vi "HoppingStep(Nonlinear-XZEnhancedSampleCurr).vi"() -> ()   [LabVIEW 2014]
uses:
  <vilib>/Platform/TimedLoop/XDataNode/timing_clust.ctl
  <vilib>/Platform/TimedLoop/XDataNode/nitl_modes.ctl
  <vilib>/Platform/TimedLoop/XDataNode/wakeup.ctl
  <vilib>/rvi/Emulation/niFpgaGetClockAttributes.vi
  <vilib>/rvi/Emulation/niFpgaSctlEmulationGetInTimedLoop.vi
  <vilib>/rvi/Emulation/niFpgaEmulationReportErrorSimple.vi
  <vilib>/rvi/Emulation/niFpgaProcessEmulError.vi
  <vilib>/rvi/eio/common/nirviEmuTemplateMethod_errors.vi
  <vilib>/rvi/Emulation/niFpgaCriticalErrorInLSC.vi
  <vilib>/rvi/interface/RandomDataEmulation/niFpgaRandomDataHandleErrors.vi
  <vilib>/eio/EIONode/EIONode.xnode
  <vilib>/Platform/TimedLoop/XDataNode/XDataNode.xnode
  <vilib>/rvi/DataTransferAndStorage/Container/XNode/niFpgaContainer.xnode
  <vilib>/rvi/interface/RandomDataEmulation/nirviRandomDataFpgaReadWriteTemplate.vi
  <vilib>/Platform/TimedLoop/XDataNode/XDNodeRunTimeDep.lvlib
panel:
  in  "ZLimitFluctuationRange":i16
  in  "CheckNum":i16
  in  "BottomSleep us":i16=80
  in  "UpperSleep us":i16=150
  out "ZRealPos":i16
  in  "RelativeWithdraw":i16
  out "Waveform Chart":i32(graph)
  in  "stop":bool
  out "Z":i32(graph)
  in  "ZOffset":i16
  in  "XOffset":i16
  in  "XNum":i16
  in  "XStepIndex":i16
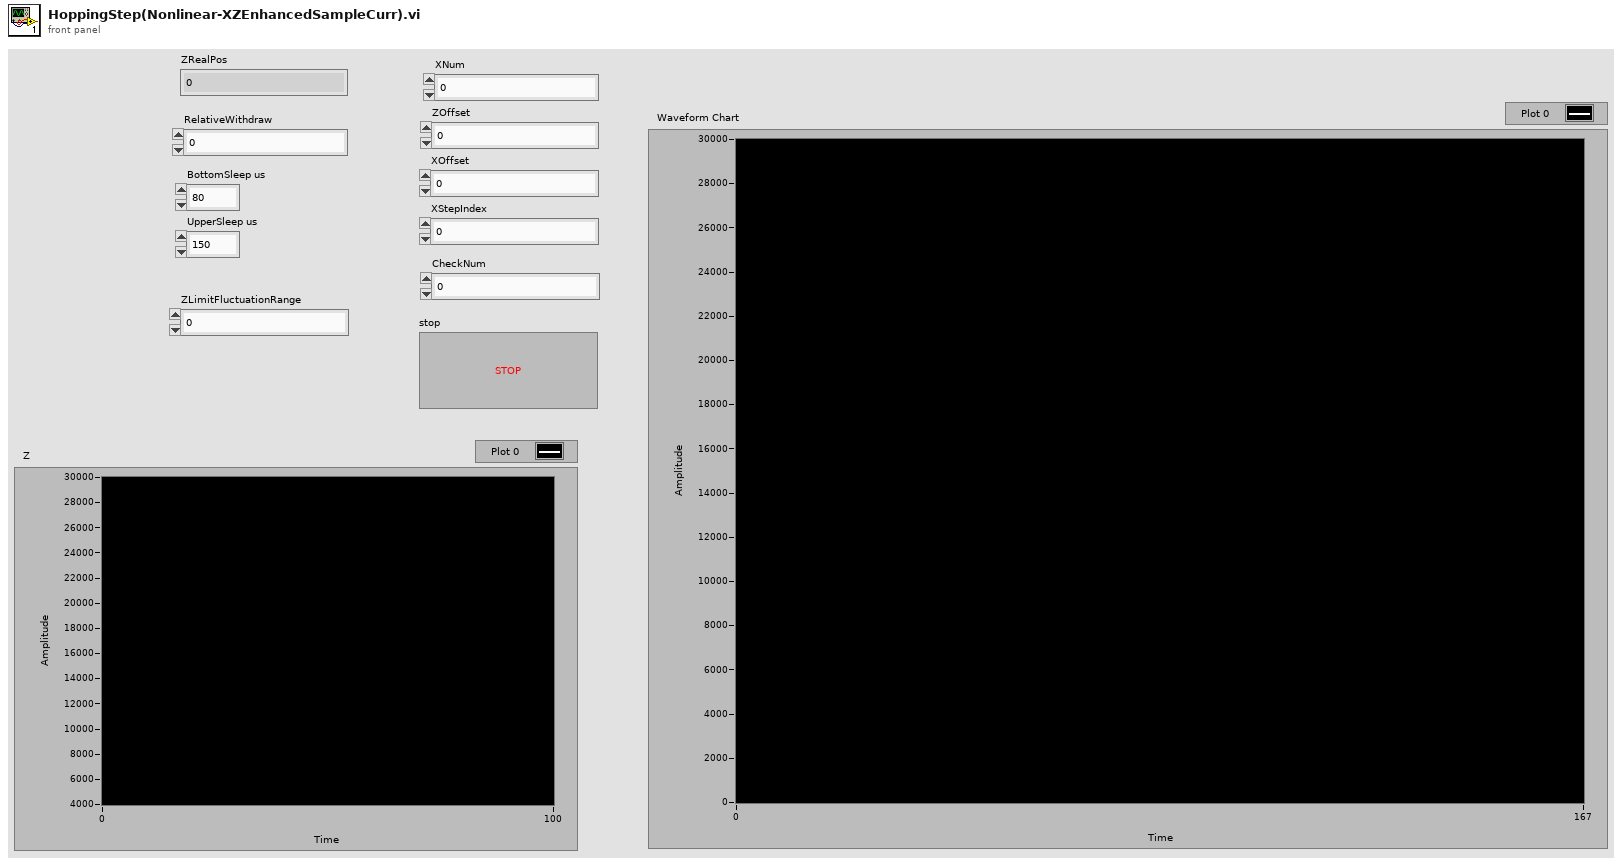
[diagram p1: front panel]
types:
  T1 = typedef "XDNodeRunTimeDep.lvlib/timing_clust.ctl" = cluster{"Expected End [f-1]":u64, "Actual End [f-1]":u64, "Finished Late? [f-1]":bool, "Expected End [i-1]":u64, "Actual End [i-1]":u64, "Finished Late? [i-1]":bool, "Expected Start [i]":u64, "Actual Start [i]":u64, "Expected Start [f]":u64, "Actual Start [f]":u64, "Source Name":string, "Structure Name":string, "Period":i64, "Deadline":i64, "Offset":i64, "Start":i64, "Priority":i32, "Timeout":i32, "Mode":T2, "Wakeup Reason":T3, "Error":errorcluster, "Source Type":string, "Secondary Source Type":string, "Global End Time":u64, "Global Start Time":u64, "Frame Duration":u64, "Iteration Duration":u64, "Assigned CPU":i32, "I/O Scan Engine Mode":u32}
  T2 = typedef "XDNodeRunTimeDep.lvlib/nitl_modes.ctl" = enum32{"No Change", "Process missed periods, maintain original phase", "Discard missed periods, maintain original phase", "Process missed periods, ignore original phase", "Discard missed periods, ignore original phase"}
  T3 = typedef "XDNodeRunTimeDep.lvlib/wakeup.ctl" = enum32{"Normal", "Aborted", "Asynchronous wakeup", "Timing source error", "Timed loop error", "Timeout"}
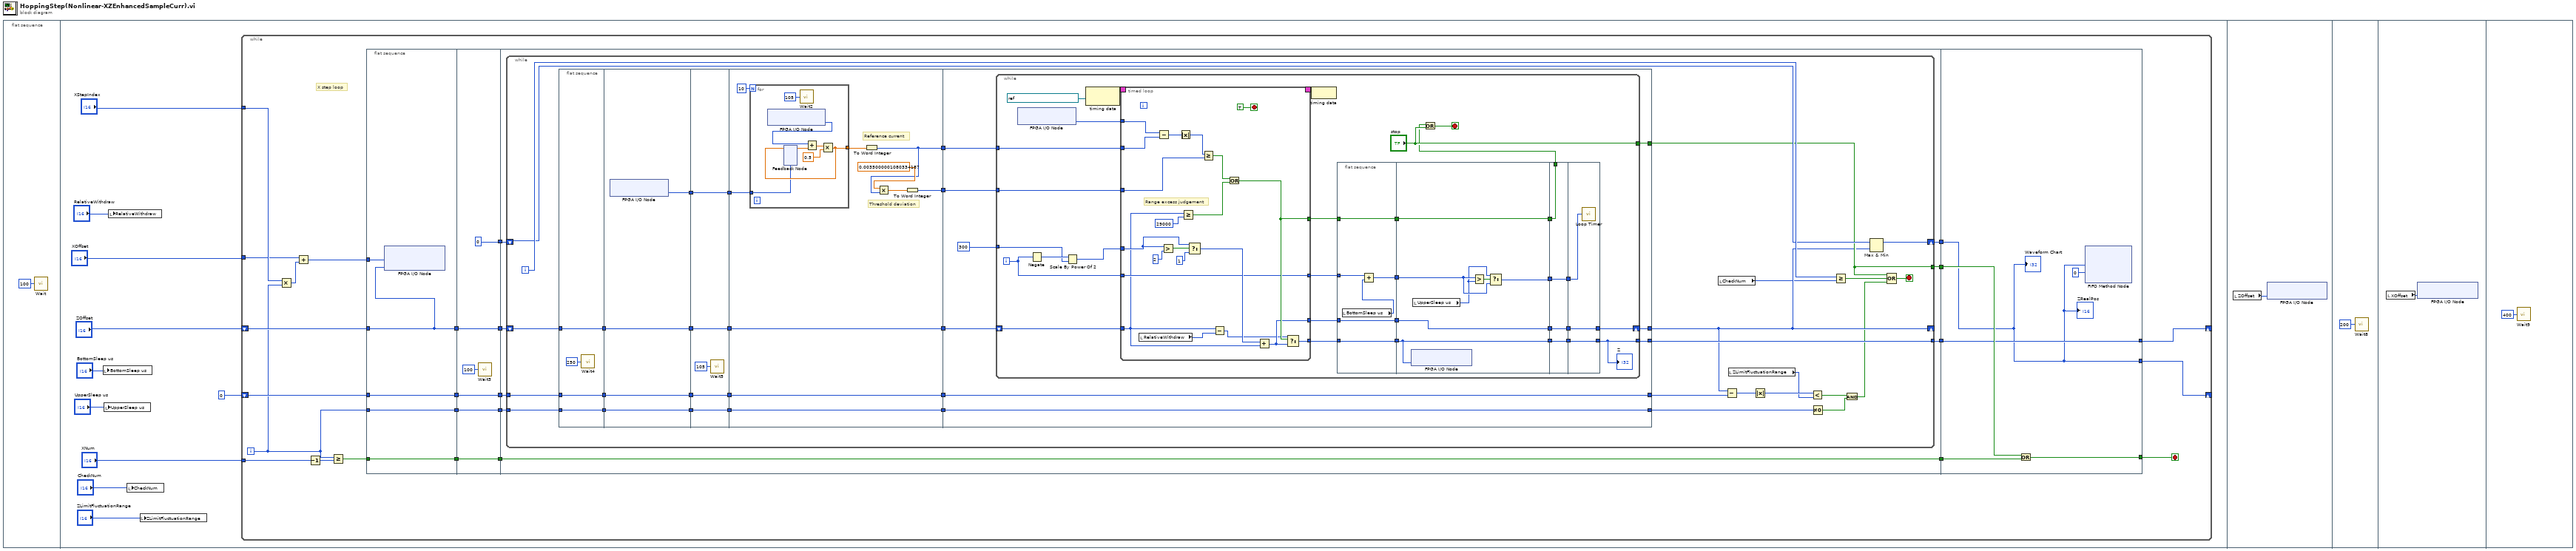
[diagram p0: block diagram]
diagram:
  n1 = flat-sequence {
    frame #0 {
      n2 = call "Wait"("Count(mSec)"=u32 100 ("Count(uSec)")) -> ()  [unwired: 1 out]
    }
    frame #1 {
      n3 = local write "BottomSleep us"("BottomSleep us") -> ()
      n4 = local write "UpperSleep us"("UpperSleep us") -> ()
      n5 = local write "RelativeWithdraw"("RelativeWithdraw") -> ()
      n6 = local write "CheckNum"("CheckNum") -> ()
      n7 = local write "ZLimitFluctuationRange"("ZLimitFluctuationRange") -> ()
      n8 = while {
        tunnel: "XNum" -> [w29]
        tunnel: "XStepIndex" -> [w30]
        shift-right: [w17] -> _
        shift-left: "ZOffset" -> [w31]
        tunnel: "XOffset" -> [w27]
        shift-right: [w16] -> _
        shift-left: i16 0 -> [w20]
        i -> [w13]
        stop <- w35 stop-if-true
        # "X step loop"
        n9 = Multiply(x=w30, y=w13) -> (x*y=w34:i32)
        n10 = Add(x=w27, y=w34) -> (x+y=w12:i32)
        n11 = Decrement(x=w29) -> (x-1=w28:i16)
        n12 = Greater Or Equal?(x=w13, y=w28) -> (x >= y?=w25:bool)
        n13 = flat-sequence {
          tunnel: [w42] -> w26
          tunnel: w31 -> [w42]
          tunnel: w25 -> [w41]
          tunnel: [w41] -> w23
          tunnel: [w40] -> w21
          tunnel: w20 -> [w40]
          tunnel: [w39] -> w14
          tunnel: w13 -> [w39]
          tunnel: w12 -> [w38]
          tunnel: [w48] -> w37
          tunnel: [i16 0] -> w33
          tunnel: w26 -> [w48]
          tunnel: [w45] -> w24
          tunnel: w23 -> [w45]
          tunnel: w21 -> [w44]
          tunnel: [w44] -> w19
          tunnel: [w43] -> w15
          tunnel: w14 -> [w43]
          tunnel: w37 -> [w56]
          tunnel: [w55] -> w36
          tunnel: w33 -> [w54]
          tunnel: [w53] -> w32
          tunnel: w24 -> [w52]
          tunnel: [w52] -> w22
          tunnel: w19 -> [w51]
          tunnel: [w50] -> w18
          tunnel: w15 -> [w49]
          tunnel: [w215] -> w35
          tunnel: w32 -> [w210]
          tunnel: w36 -> [w213]
          tunnel: w22 -> [w212]
          tunnel: w18 -> [w211]
          tunnel: [w211] -> w17
          tunnel: [w210] -> w16
          frame #0 {
            n14 = xnode "FPGA I/O Node"("Connector0/AO2"=w38, "Connector0/AO0"=w42) -> ()  [unwired: 2 in, 2 out]
          }
          frame #1 {
            n15 = call "Wait3"("Count(uSec)"=u32 100) -> ()  [unwired: 1 out]
          }
          frame #2 {
            n16 = while {
              tunnel: [w70] -> w55
              shift-right: [w69] -> _
              shift-left: w56 -> [w89]
              shift-right: [w90] -> w53
              shift-left: w54 -> [w91]
              tunnel: w51 -> [w80]
              tunnel: [w77] -> w50
              tunnel: w49 -> [w76]
              i -> [w92]
              stop <- w72 stop-if-true
              n17 = flat-sequence {
                tunnel: w76 -> [w94]
                tunnel: w80 -> [w95]
                tunnel: w89 -> [w96]
                tunnel: [w96] -> w59
                tunnel: [w95] -> w58
                tunnel: [w94] -> w57
                tunnel: [w100] -> w84
                tunnel: [w99] -> w82
                tunnel: [w98] -> w81
                tunnel: [w97] -> w74
                tunnel: w59 -> [w100]
                tunnel: w58 -> [w98]
                tunnel: w57 -> [w97]
                tunnel: [w105] -> w85
                tunnel: w84 -> [w105]
                tunnel: [w103] -> w83
                tunnel: w82 -> [w103]
                tunnel: w81 -> [w102]
                tunnel: [w102] -> w78
                tunnel: [w101] -> w75
                tunnel: w74 -> [w101]
                tunnel: [w109] -> w88
                tunnel: [w108] -> w87
                tunnel: [w115] -> w86
                tunnel: w85 -> [w115]
                tunnel: w83 -> [w113]
                tunnel: [w107] -> w79
                tunnel: w78 -> [w107]
                tunnel: w75 -> [w106]
                tunnel: [w106] -> w73
                tunnel: [w129] -> w70
                tunnel: [w128] -> w69
                tunnel: w88 -> [w131]
                tunnel: w87 -> [w130]
                tunnel: w86 -> [w126]
                tunnel: w79 -> [w125]
                tunnel: [w125] -> w68
                tunnel: [w124] -> w77
                tunnel: w73 -> [w123]
                tunnel: [w123] -> w64
                frame #0 {
                  n18 = call "Wait4"("Count(uSec)"=u32 250) -> ()  [unwired: 1 out]
                }
                frame #1 {
                  n19 = xnode "FPGA I/O Node"() -> ("Connector0/AI1"=w99:i16)  [unwired: 1 in, 1 out]
                }
                frame #2 {
                  n20 = call "Wait5"("Count(uSec)"=u32 105) -> ()  [unwired: 1 out]
                }
                frame #3 {
                  # "Threshold deviation"
                  # "Reference current"
                  n21 = for {
                    N: 10 -> [_]
                    tunnel: [w117] -> w110
                    tunnel: w113 -> [w116]
                    n22 = xnode "FPGA I/O Node"() -> ("Connector0/AI1"=w118:i16)  [unwired: 1 in, 1 out]
                    n23 = feedback #1(w116) -> (w121:sgl)
                    n24 = call "Wait2"("Count(uSec)"=u32 105) -> ()  [unwired: 1 out]
                    n25 = Add(x=w118, y=w121) -> (x+y=w120:sgl)
                    n26 = Multiply(x=w120, y=sgl 0.5) -> (x*y=w117:sgl)
                    n27 = feedback-in #1(w117) -> ()
                  }
                  n28 = To Word Integer(number=w110) -> (16bit integer=w109:i16)
                  n29 = Multiply(x=sgl 0.0035, y=w109) -> (x*y=w111:sgl)
                  n30 = To Word Integer(number=w111) -> (16bit integer=w108:i16)
                }
                frame #4 {
                  n31 = while {
                    tunnel: w131 -> [w155]
                    tunnel: w130 -> [w157]
                    tunnel: ["stop"] -> w129
                    shift-right: [w147] -> w128
                    shift-left: w126 -> [w152]
                    tunnel: i16 300 -> [w137]
                    tunnel: [w132] -> w124
                    i -> [w135]
                    stop <- w159 stop-if-true
                    n32 = xnode "FPGA I/O Node"() -> ("Connector0/AI1"=w156:i16)  [unwired: 1 in, 1 out]
                    n33 = Negate(x=w135) -> (-x=w138:i32)
                    n34 = Scale By Power Of 2(n=w138, x=w137) -> (x*2^n=w136:i16)
                    n35 = node-c288(refnum<k21> "40 MHz Onboard Clock" ("Source Name")) -> (w162:T1)
                    n36 = timed-loop {
                      timing: w162 -> [_]
                      timing-out: [_] -> w161
                      tunnel: w155 -> [w201]
                      tunnel: w157 -> [w186]
                      tunnel: w156 -> [w202]
                      tunnel: [w197] -> w153
                      tunnel: [w196] -> w151
                      tunnel: w152 -> [w185]
                      tunnel: [w194] -> w149
                      tunnel: w136 -> [w189]
                      tunnel: [w191] -> w139
                      tunnel: w135 -> [w191]
                      stop <- TRUE stop-if-true
                      # "Range excess judgement"
                      n37 = local read "RelativeWithdraw"() -> (w183:i16)
                      n38 = Subtract(x=w202, y=w201) -> (x-y=w187:i16)
                      n39 = Greater?(x=w189, y=i16 2) -> (0:w188:bool)
                      n40 = Absolute Value(x=w187) -> (abs(x)=w200:i16)
                      n41 = Greater Or Equal?(x=w185, y=i16 29000) -> (x >= y?=w198:bool)
                      n42 = Select(t=w189, s=w188, f=1) -> (s? t:f=w192:i32)
                      n43 = Greater Or Equal?(x=w200, y=w186) -> (x >= y?=w199:bool)
                      n44 = Subtract(x=w185, y=w183) -> (x-y=w184:i32)
                      n45 = Or(x=w199, y=w198) -> (x .or. y?=w196:bool)
                      n46 = Add(x=w192, y=w185) -> (x+y=w194:i32)
                      n47 = Select(t=w184, s=w196, f=w194) -> (s? t:f=w197:i32)
                    }
                    n48 = node-c288(w161) -> ()
                    n49 = flat-sequence {
                      tunnel: [w168] -> w154
                      tunnel: w153 -> [w168]
                      tunnel: w151 -> [w167]
                      tunnel: [w167] -> w150
                      tunnel: w149 -> [w166]
                      tunnel: [w166] -> w148
                      tunnel: [w164] -> w140
                      tunnel: w139 -> [w165]
                      tunnel: w154 -> [w169]
                      tunnel: [w175] -> w146
                      tunnel: w150 -> [w174]
                      tunnel: w148 -> [w175]
                      tunnel: [w174] -> w144
                      tunnel: [w172] -> w141
                      tunnel: w140 -> [w171]
                      tunnel: [w169] -> w133
                      tunnel: w146 -> [w179]
                      tunnel: [w179] -> w145
                      tunnel: w144 -> [w178]
                      tunnel: [w178] -> w143
                      tunnel: [w177] -> w142
                      tunnel: w141 -> [w177]
                      tunnel: [w176] -> w134
                      tunnel: w133 -> [w176]
                      tunnel: w145 -> [w182]
                      tunnel: [w182] -> w147
                      tunnel: w142 -> [w181]
                      tunnel: [w180] -> w132
                      tunnel: w134 -> [w180]
                      frame #0 {
                        n50 = local read "BottomSleep us"() -> (w163:i16)
                        n51 = Add(x=w165, y=w163) -> (x+y=w164:i32)
                      }
                      frame #1 {
                        n52 = xnode "FPGA I/O Node"("Connector0/AO0"=w169) -> ()  [unwired: 1 in, 1 out]
                        n53 = local read "UpperSleep us"() -> (w170:i16)
                        n54 = Greater?(x=w171, y=w170) -> (0:w173:bool)
                        n55 = Select(t=w170, s=w173, f=w171) -> (s? t:f=w172:i32)
                      }
                      frame #2 {
                      }
                      frame #3 {
                        n56 = call "Loop Timer"("Count(uSec)"=w181) -> ()  [unwired: 1 out]
                      }
                    }
                    n57 = Or(x=w143, y="stop") -> (x .or. y?=w159:bool)
                    "Z" <- w132
                  }
                }
              }
              n58 = local read "CheckNum"() -> (w60:i16)
              n59 = Subtract(x=w69, y=w68) -> (x-y=w67:i32)
              n60 = local read "ZLimitFluctuationRange"() -> (w65:i16)
              n61 = Absolute Value(x=w67) -> (abs(x)=w66:i32)
              n62 = Less?(x=w66, y=w65) -> (x < y?=w63:bool)
              n63 = Not Equal To 0?(x=w64) -> (x != 0?=w62:bool)
              n64 = Greater Or Equal?(x=w92, y=w60) -> (x >= y?=w71:bool)
              n65 = And(x=w63, y=w62) -> (x .and. y?=w61:bool)
              n66 = Max & Min(x=w91, y=w69) -> (max(x,y)=w90:i32)  [unwired: 1 out]
              n67 = Compound Arithmetic op=OR(w70, w71, w61) -> (w72:bool)
            }
          }
          frame #3 {
            n68 = Or(x=w213, y=w212) -> (x .or. y?=w215:bool)
            n69 = xnode ("FIFO Method Node")("Element"=w210, "Timeout"=0) -> ()  [unwired: 1 in, 2 out]
            "Waveform Chart" <- w210
            "ZRealPos" <- w210
          }
        }
      }
    }
    frame #2 {
      n70 = local read "ZOffset"() -> (w216:i16)
      n71 = xnode "FPGA I/O Node"("Connector0/AO0"=w216) -> ()  [unwired: 1 in, 1 out]
    }
    frame #3 {
      n72 = call "Wait8"("Count(uSec)"=u32 200) -> ()  [unwired: 1 out]
    }
    frame #4 {
      n73 = local read "XOffset"() -> (w218:i16)
      n74 = xnode "FPGA I/O Node"("Connector0/AO2"=w218) -> ()  [unwired: 1 in, 1 out]
    }
    frame #5 {
      n75 = call "Wait9"("Count(uSec)"=u32 400) -> ()  [unwired: 1 out]
    }
  }
